vi "Example 1.vi"   [LabVIEW 2018]
uses:
  <vilib>/addons/VeriStand Custom Device Scripting APIs/FPGA Addon/Scripting API.lvlibp/APIs/Scripting API/Private/Import Bitfile Scalars (Instances)/Import Scalars - all.vi
  <vilib>/addons/VeriStand Custom Device Scripting APIs/FPGA Addon/Scripting API.lvlibp
types:
  T1 = typedef "Scripting API.lvlibp/Custom Device API.lvlib/Custom Device Item Ref.ctl" = u64
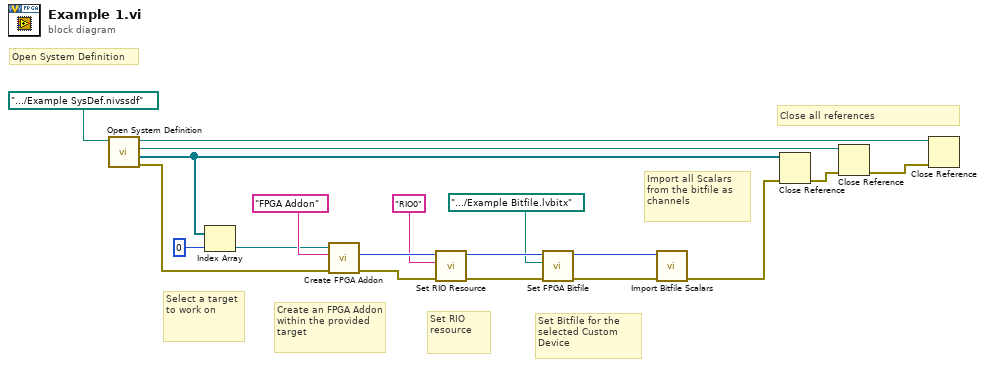
[diagram p0: block diagram]
diagram:
  # "Close all references"
  # "Import all Scalars from the bitfile as channels"
  # "Set Bitfile for the selected Custom Device"
  # "Set RIO resource"
  # "Create an FPGA Addon within the provided target"
  # "Select a target to work on"
  # "Open System Definition"
  n1 = call "Open System Definition.vi"("System Definition File"=path ".../Example SysDef.nivssdf" ("fpga bitfile path")) -> ("error out"=w12:errorcluster, "targets refnums"=w15:refnum<k24>[], "root refnum"=w16:refnum<k24>, "system definition refnum"=w17:refnum<k24>)  [unwired: 7 in]
  n2 = Index Array(array=w15, index=0) -> (element=w10:refnum<k24>)
  n3 = call <vilib>:"Create FPGA Addon.vi"("error in (no error)"=w12, "FPGA Addon name"="FPGA Addon" ("fpga addon name"), "target in"=w10) -> ("error out"=w9:errorcluster, "FPGA Addon refnum"=w8:T1)  [unwired: 6 in, 1 out]
  n4 = call <vilib>:"Set RIO Resource.vi"("error in (no error)"=w9, "rio resource in"="RIO0", "FPGA Addon refnum in"=w8) -> ("error out"=w6:errorcluster, "FPGA Addon refnum out"=w5:T1)  [unwired: 7 in]
  n5 = call <vilib>:"Set FPGA Bitfile.vi"("error in (no error)"=w6, "fpga bitfile path"=path ".../Example Bitfile.lvbitx", "FPGA Addon refnum in"=w5) -> ("error out"=w2:errorcluster, "FPGA Addon refnum out"=w3:T1)  [unwired: 7 in]
  n6 = call-poly <vilib>:"Import Bitfile Scalars.vi"("error in (no error)"=w2, "FPGA Addon refnum in"=w3) -> ("error out"=w1:errorcluster)  [unwired: 7 in, 2 out]
  n7 = Close Reference(reference=w15, error in (no error)=w1) -> (error out=w14:errorcluster)
  n8 = Close Reference(reference=w16, error in (no error)=w14) -> (error out=w13:errorcluster)
  n9 = Close Reference(reference=w17, error in (no error)=w13) -> ()  [unwired: 1 out]
